vi "LeerBD.vi"(8 "error in (no error)":errorcluster) -> (0 "error out":errorcluster, 2 "BD":T1={"MaxNivelCpeak"=97.0, "Incertidumbre"=[], "Tol +"=[], "Tol -"=[]}, 3 "Prueba09 out":refnum<class "Prueba09.lvclass">)   [LabVIEW 2019, in "Prueba09.lvclass"]
uses:
  Prueba09.lvclass
  BD.ctl
  Base de Datos/SQLiteConnector/SQLiteConnection.lvclass
  Base de Datos/Base de Datos.lvclass
panel:
  in  "Tipo Equipo":enum16{"Sonometro", "Calibrador", "Dosimetro"}(ring)
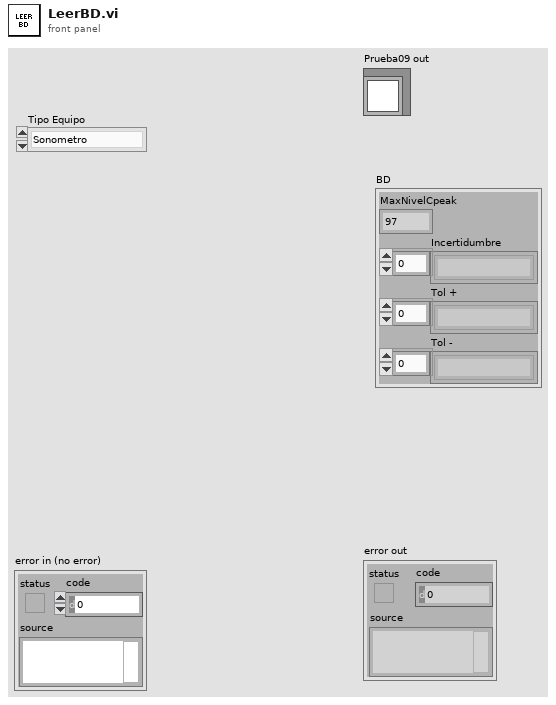
[diagram p1: front panel]
types:
  T1 = typedef "Prueba09.lvclass/BD.ctl" = cluster{"MaxNivelCpeak":dbl, "Incertidumbre":string[], "Tol +":string[], "Tol -":string[]}
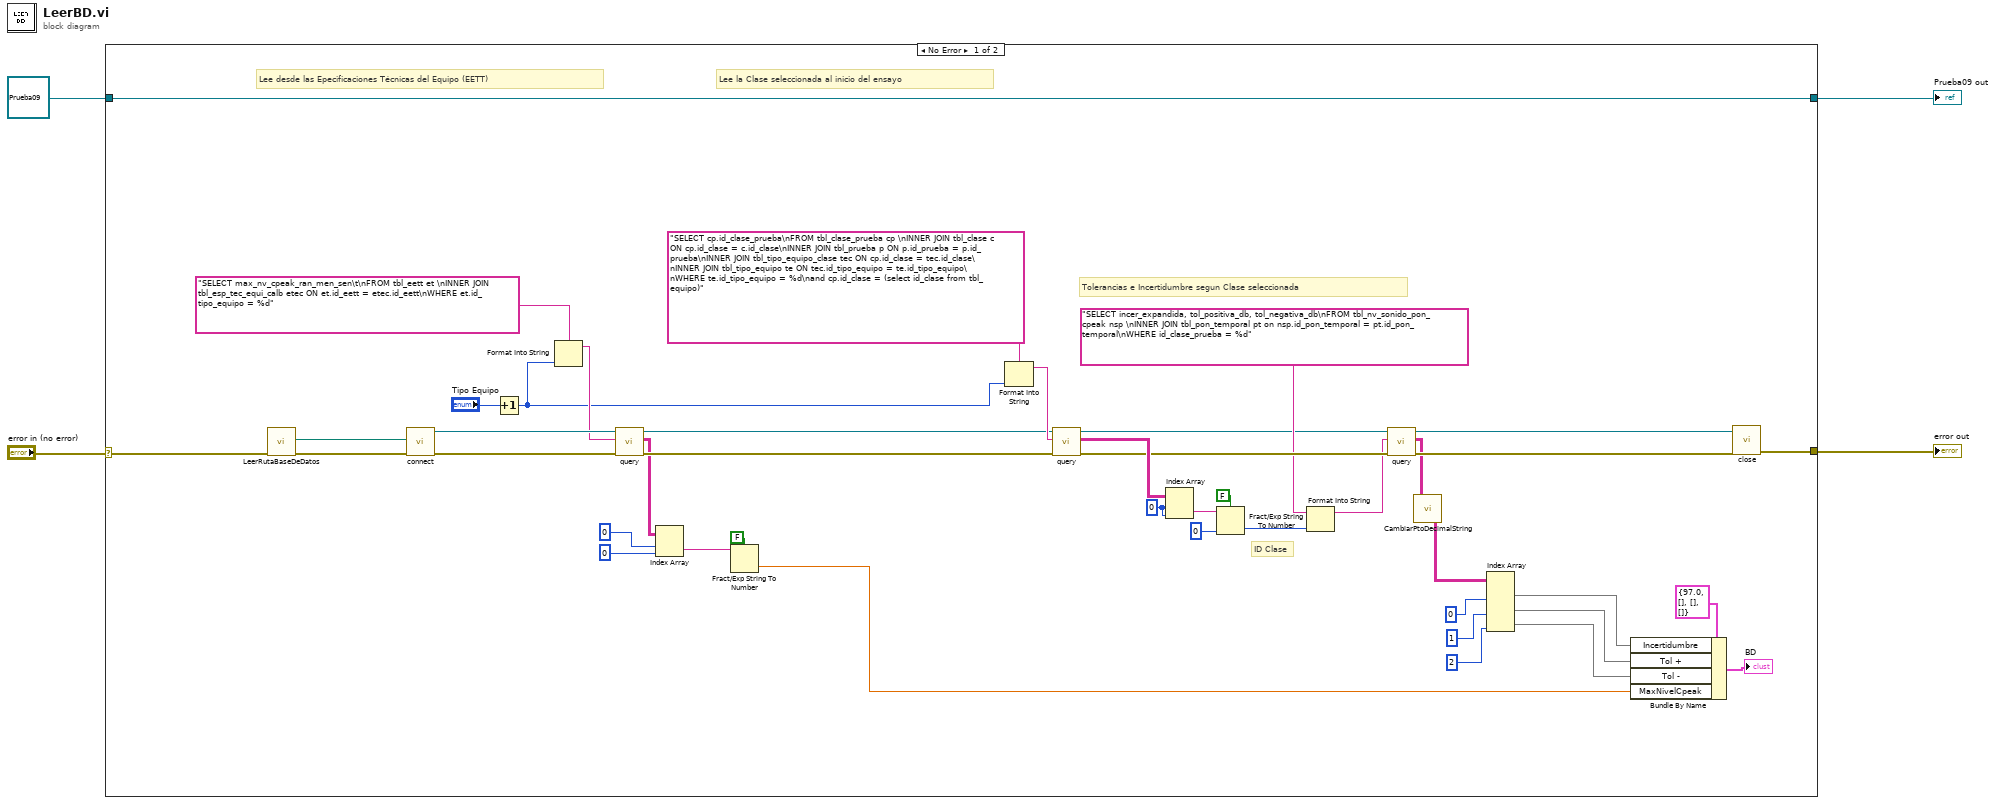
[diagram p0: block diagram]
diagram:
  n1 = case shown="No Error" "error in (no error)" {
    selector: "error in (no error)" -> [w39 w49]
    tunnel: [w25 w49] -> w3
    tunnel: [w47 w48] -> w1
    tunnel: refnum<class "Prueba09.lvclass"> refnum ("Prueba02 in") -> [w47 w48]
    frame No Error {
      w31 = 0 ("index (row)")
      # "Tolerancias e Incertidumbre segun Clase seleccionada"
      # "ID Clase"
      # "Lee la Clase seleccionada al inicio del ensayo"
      # "Lee desde las Epecificaciones Técnicas del Equipo (EETT)"
      n2 = call "LeerRutaBaseDeDatos.vi"("error in (no error)"=w39) -> ("error out"=w42:errorcluster, "Database Path"=w41:path)  [unwired: 9 in]
      n3 = call "connect.vi"("error in (no error)"=w42, "Database Path"=w41) -> ("error out"=w44:errorcluster, "object out"=w45:refnum<class "SQLiteConnection.lvclass">)  [unwired: 8 in]
      n4 = Increment(x="Tipo Equipo") -> (x+1=w20:enum16{"Sonometro", "Calibrador", "Dosimetro"})
      n5 = Format Into String(format string="SELECT max_nv_cpeak_ran_men_sen\t\nFROM tbl_eett et \nINNER JOIN tbl_esp_tec_equi_calb etec ON et.id_eett = etec.id_eett\nWHERE et.id_tipo_equipo = %d", w20) -> (resulting string=w43:string)  [unwired: 2 in, 1 out]
      n6 = call "query.vi"("error in (no error)"=w44, "SQL Statement"=w43, "object in"=w45) -> ("error out"=w32:errorcluster, "result"=w13:string[][], "object out"=w33:refnum<class "SQLiteConnection.lvclass">)  [unwired: 5 in, 1 out]
      n7 = Index Array(array=w13, index (row)=0, index (col)=0 ("disabled index (col)")) -> (element=w37:string)
      n8 = Fract/Exp String To Number(use system decimal point (T)=FALSE, string=w37) -> (number=w6:dbl)  [unwired: 2 in, 1 out]
      n9 = Format Into String(format string="SELECT cp.id_clase_prueba\nFROM tbl_clase_prueba cp \nINNER JOIN tbl_clase c ON cp.id_clase = c.id_clase\nINNER JOIN tbl_prueba p ON p.id_prueba = p.id_prueba\nINNER JOIN tbl_tipo_equipo_clase tec ON cp.id_clase = tec.id_clase\nINNER JOIN tbl_tipo_equipo te ON tec.id_tipo_equipo = te.id_tipo_equipo\nWHERE te.id_tipo_equipo = %d\nand cp.id_clase = (select id_clase from tbl_equipo)", w20) -> (resulting string=w34:string)  [unwired: 2 in, 1 out]
      n10 = call "query.vi"("error in (no error)"=w32, "SQL Statement"=w34, "object in"=w33) -> ("error out"=w26:errorcluster, "result"=w27:string[][], "object out"=w22:refnum<class "SQLiteConnection.lvclass">)  [unwired: 5 in, 1 out]
      n11 = Index Array(array=w27, index (row)=w31, index (col)=w31) -> (element=w29:string)
      n12 = Fract/Exp String To Number(use system decimal point (T)=FALSE, string=w29, default (0 dbl)=0 ("index (row)")) -> (number=w17:i32)  [unwired: 1 in, 1 out]
      n13 = Format Into String(format string="SELECT incer_expandida, tol_positiva_db, tol_negativa_db\nFROM tbl_nv_sonido_pon_cpeak nsp \nINNER JOIN tbl_pon_temporal pt on nsp.id_pon_temporal = pt.id_pon_temporal\nWHERE id_clase_prueba = %d", w17) -> (resulting string=w21:string)  [unwired: 2 in, 1 out]
      n14 = call "query.vi"("error in (no error)"=w26, "SQL Statement"=w21, "object in"=w22) -> ("error out"=w23:errorcluster, "result"=w19:string[][], "object out"=w18:refnum<class "SQLiteConnection.lvclass">)  [unwired: 5 in, 1 out]
      n15 = call "CambiarPtoDecimalString.vi"("result"=w19) -> ("result out"=w5:string[][])
      n16 = Index Array(array=w5, index (col) #1=0 ("disabled index (col)"), index (col) #2=1 ("disabled index (col)"), index (col) #3=2 ("disabled index (col)")) -> (element #1=w9:string[], element #2=w8:string[], element #3=w7:string[])  [unwired: 3 in]
      n17 = Bundle By Name(cluster=T1 {"MaxNivelCpeak"=97.0, "Incertidumbre"=[], "Tol +"=[], "Tol -"=[]} ("BD"), "Incertidumbre"=w9, "Tol +"=w8, "Tol -"=w7, "MaxNivelCpeak"=w6) -> (→"BD":T1)
      n18 = call-dynamic "close.vi"("error in (no error)"=w23, "object in"=w18) -> ("error out"=w25:errorcluster)  [unwired: 8 in, 1 out]
    }
    frame Error {
    }
  }
  "error out" <- w3
  "Prueba09 out" <- w1
